vi "testInvalidRefnum.vi"() -> (0 "error out":errorcluster)   [LabVIEW 2017, in "Fact.Tests.lvlib"]
uses:
  Fact.Tests.lvlib
  Fact/Fact.lvclass
  Assertion/Assertion.lvlib
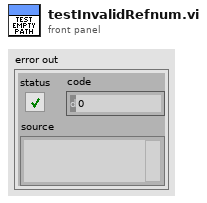
[diagram p1: front panel]
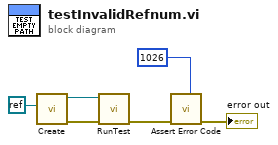
[diagram p0: block diagram]
diagram:
  n1 = call "Create.vi"("VI Refnum"=refnum<k0> refnum) -> ("error out"=w5:errorcluster, "Fact"=w6:refnum<class "Fact.lvclass">)  [unwired: 9 in]
  n2 = call-dynamic "RunTest.vi"("error in (no error)"=w5, "Fact in"=w6) -> ("error out"=w4:errorcluster)  [unwired: 8 in, 1 out]
  n3 = call "Assert Error Code.vi"("Expected"=1026, "error in (no error)"=w4) -> ("error out"=→"error out":errorcluster)  [unwired: 9 in]
